vi "xI32 To XML.vi"(1 "variable":i32, 2 "variable name":string="test") -> (0 "xml string":string)   [LabVIEW 2012]
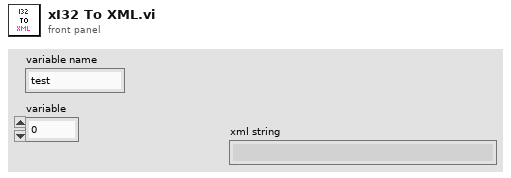
[diagram p1: front panel]
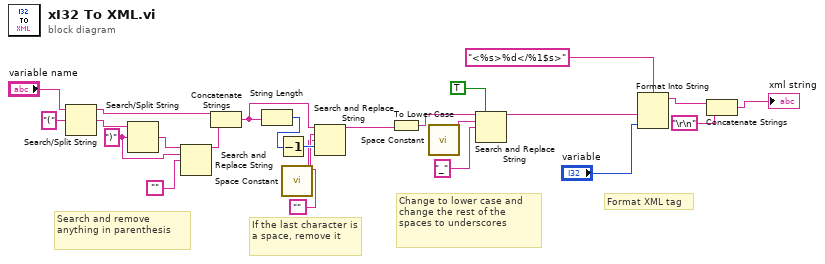
[diagram p0: block diagram]
diagram:
  w8 = ")" ("search string/char (-)")
  # "Format XML tag"
  # "Change to lower case and change the rest of the spaces to underscores"
  # "If the last character is a space, remove it"
  # "Search and remove anything in parenthesis"
  n1 = Search/Split String(string="variable name", search string/char (-)="(") -> (substring before match=w12:string, match + rest of string=w13:string)  [unwired: 1 in, 1 out]
  n2 = Search/Split String(string=w13, search string/char (-)=w8) -> (match + rest of string=w10:string)  [unwired: 1 in, 2 out]
  n3 = Search and Replace String(input string=w10, search string=w8, replace string="") -> (result string=w7:string)  [unwired: 5 in, 3 out]
  n4 = Concatenate Strings(w12, w7) -> (w4:string)
  n5 = String Length(string=w4) -> (length=w6:i32)
  n6 = Decrement(x=w6) -> (x-1=w5:i32)
  n7 = call <vilib>:"Space Constant.vi"() -> ("String"=w3:string)
  n8 = Search and Replace String(input string=w4, search string=w3, replace string="", offset=w5) -> (result string=w1:string)  [unwired: 4 in, 3 out]
  n9 = To Lower Case(string=w1) -> (all lower case string=w19:string)
  n10 = call <vilib>:"Space Constant.vi"() -> ("String"=w17:string)
  n11 = Search and Replace String(replace all?=TRUE ("replace all? (F)"), input string=w19, search string=w17, replace string="_") -> (result string=w15:string)  [unwired: 4 in, 3 out]
  n12 = Format Into String(format string="<%s>%d</%1$s>" ("format string (<%s>%d</%1$s>)"), w15, "variable") -> (resulting string=w22:string)  [unwired: 2 in, 1 out]
  n13 = Concatenate Strings(w22, "\r\n") -> (→"xml string":string)
